vi "ROI entry-ROI within img boundary.vi"(11 "Coordinates in":i32[](array[numeric])) -> (3 "Coordinates out":i32[](array[numeric]))   [LabVIEW 2013]
panel:
  # "X1\nY1\nX2\nY2"
  # "X1\nY1\nX2\nY2"
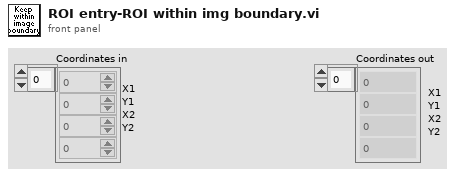
[diagram p1: front panel]
types:
  T1 = typedef "IMAQ Image.ctl" = refnum<image>
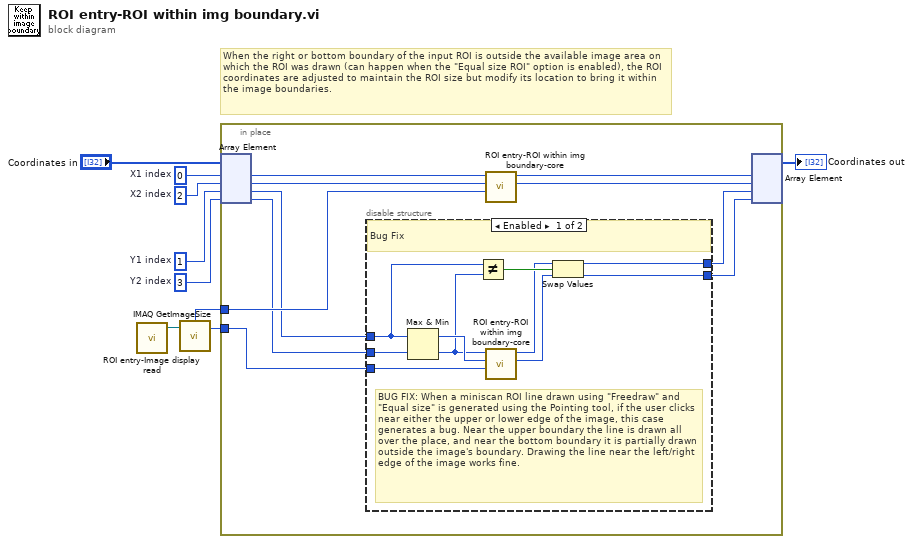
[diagram p0: block diagram]
diagram:
  w2 = 1  # Y1 index
  w9 = 0  # X1 index
  w1 = 3  # Y2 index
  w4 = 2  # X2 index
  # "When the right or bottom boundary of the input ROI is outside the available image area on which the ROI was drawn (can happen when the \"Equal size ROI\" option is enabled), the ROI coordinates are adjusted to maintain the ROI size but modify its location to bring it within the image boundaries."
  n1 = call "ROI entry-Image display read.vi"() -> ("CurrentImage"=w7:T1)  [unwired: 4 in, 1 out]
  n2 = call "IMAQ GetImageSize"("Image"=w7) -> ("Y Resolution"=w5:i32, "X Resolution"=w6:i32)  [unwired: 3 in, 1 out]
  n3 = in-place {
    in-place-border: w6 -> [w17]
    in-place-border: w5 -> [w14]
    n4 = in-place-array #1("Coordinates in", w9, w4, w2, w1) -> (w19:i32, w16:i32, w12:i32, w13:i32)
    n5 = disable-structure shown="Enabled" {
      disable-tunnel: w14 -> [w29 _]
      disable-tunnel: w13 -> [w28 w30]
      disable-tunnel: w12 -> [w25 w31]
      disable-tunnel: [w21 w31] -> w11
      disable-tunnel: [w20 w30] -> w10
      frame Enabled {
        # "BUG FIX: When a miniscan ROI line drawn using \"Freedraw\" and \"Equal size\" is generated using the Pointing tool, if the user clicks near either the upper or lower edge of the image, this case generates a bug. Near the upper boundary the line is drawn all over the place, and near the bottom boundary it is partially drawn outside the image's boundary. Drawing the line near the left/right edge of the image works fine."
        # "Bug Fix"
        n6 = Max & Min(x=w25, y=w28) -> (max(x,y)=w27:i32, min(x,y)=w26:i32)
        n7 = Not Equal?(x=w25, y=w26) -> (x != y?=w24:bool)
        n8 = call "ROI entry-ROI within img boundary-core.vi"("Image resolution"=w29, "ROI Max (zero based)"=w27, "ROI Min (zero based)"=w26) -> ("ROI Max"=w22:i32, "ROI Min"=w23:i32)  [unwired: 7 in]
        n9 = Swap Values(12:w23, 13:w24, 14:w22) -> (1:w21:i32, 3:w20:i32)
      }
      frame Disabled {
      }
    }
    n10 = call "ROI entry-ROI within img boundary-core.vi"("Image resolution"=w17, "ROI Max (zero based)"=w16, "ROI Min (zero based)"=w19) -> ("ROI Max"=w15:i32, "ROI Min"=w18:i32)  [unwired: 7 in]
    n11 = in-place-array #1(w18, w15, w11, w10) -> (→"Coordinates out":i32[])  [unwired: 4 out]
  }
